vi "TCPC.vi"(11 "data out":string) -> (3 "offset past number":dbl format="%#_3f")   [LabVIEW 2014]
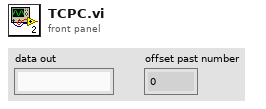
[diagram p1: front panel]
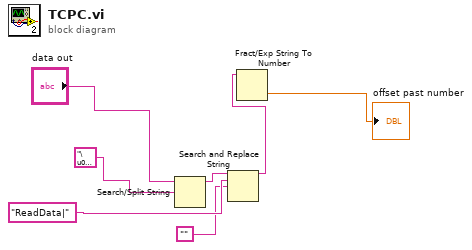
[diagram p0: block diagram]
diagram:
  n1 = Search/Split String(string="data out", search string/char (-)="\u0000") -> (substring before match=w6:string)  [unwired: 1 in, 2 out]
  n2 = Search and Replace String(input string=w6, search string="ReadData|" ("搜索字符串/字符(-)"), replace string="") -> (result string=w3:string)  [unwired: 5 in, 3 out]
  n3 = Fract/Exp String To Number(string=w3) -> (number=→"offset past number":dbl)  [unwired: 3 in, 1 out]
